vi "CFTS-Connections Dialog.vi"(2 "Parent VI":refnum<vi>) -> ()   [LabVIEW 2020]
doc: "Use this template to create a dialog box with event handling."
uses:
  epl-vi-lib/Utility VIs/Controls/KBackground Gradient/KBackground Gradient.xctl
  epl-vi-lib/Utility VIs/Controls/KTable/KTable.xctl
  epl-vi-lib/Connection VIs/Typedefs/CM-Endpoint.ctl
panel:
  in  "AO":u16(xcontrol)
  in  "AI":u16(xcontrol)
  in  "background":dbl(xcontrol)
  in  "Cancel":bool
  in  "OK":bool
  # "Connections"
  # "Outputs"
  # "Inputs"
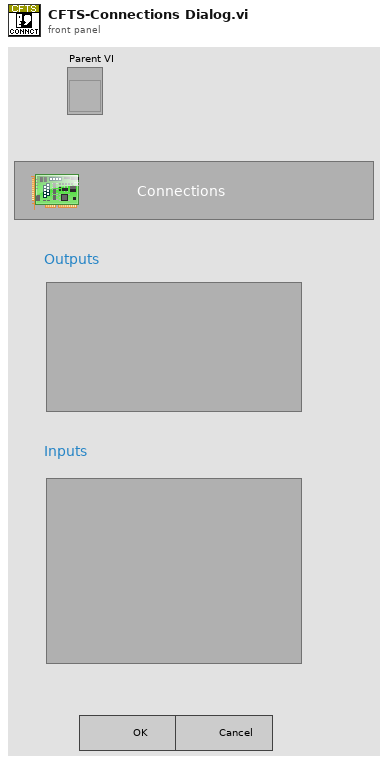
[diagram p1: front panel]
types:
  T1 = typedef "CM-Endpoint.ctl" = cluster{"Name":string, "Device":string}
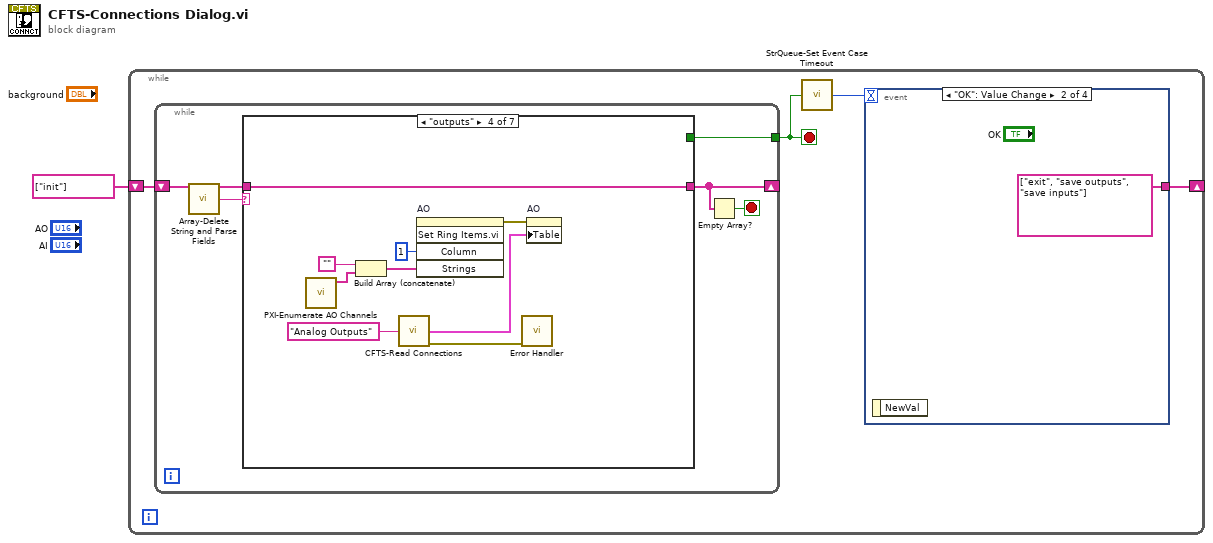
[diagram p0: block diagram]
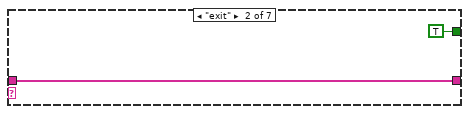
[diagram p3: hidden frame]
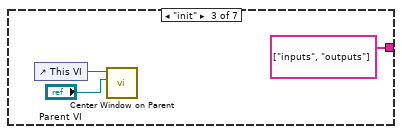
[diagram p4: hidden frame]
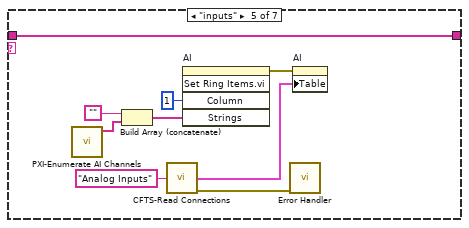
[diagram p5: hidden frame]
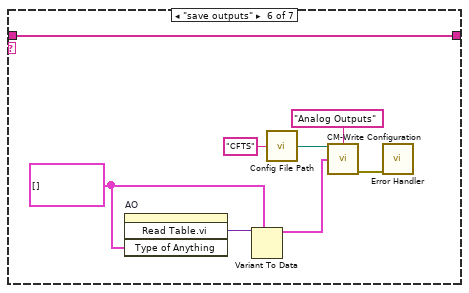
[diagram p6: hidden frame]
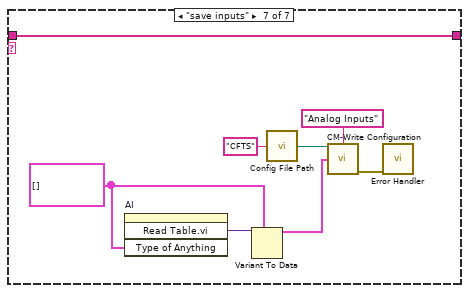
[diagram p7: hidden frame]
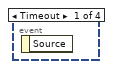
[diagram p8: hidden frame]
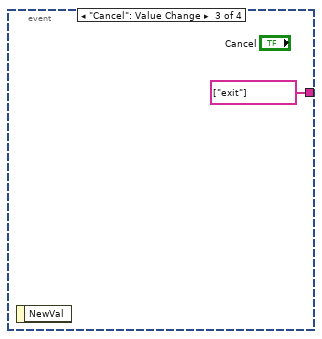
[diagram p9: hidden frame]
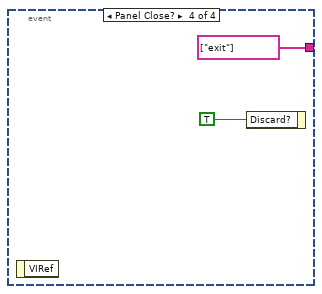
[diagram p10: hidden frame]
diagram:
  n1 = while {
    shift-right: [w2] -> _
    shift-left: string[] ["init"] -> [w3]
    stop <- w5 stop-if-true
    n2 = while {
      shift-right: [w11] -> _
      shift-left: w3 -> [w8]
      tunnel: [w9] -> w5
      stop <- w10 stop-if-true
      n3 = call "Array-Delete String and Parse Fields.vi"("Array in"=w8) -> ("Array out"=w7:string[], "Field 1"=w6:string)  [unwired: 10 in, 3 out]
      n4 = case shown="\"outputs\"" w6 {
        tunnel: w7 -> [w12 w14 _ w26 w35 w43 w51]
        tunnel: [w12 w14 string[] ["inputs", "outputs"] ("Array out") w26 w35 w43 w51] -> w11
        tunnel: [_ TRUE _ _ _ _ _] -> w9
        frame "", Default {
        }
        frame "exit" {
        }
        frame "init" {
          n5 = control-ref of="This VI"() -> (w16:refnum<vi>)
          n6 = call "Center Window on Parent.vi"("Parent VI"="Parent VI", "VI in"=w16) -> ()  [unwired: 8 in, 2 out]
        }
        frame "outputs" {
          n7 = call "PXI-Enumerate AO Channels.vi"() -> ("AO.PhysicalChans"=w23:tag[])  [unwired: 11 in]
          n8 = Build Array (concatenate)("", w23) -> (w21:string[])
          n9 = call "CFTS-Read Connections.vi"("Which"="Analog Outputs") -> ("endpoints"=w19:T1[], "error out"=w20:errorcluster)  [unwired: 13 in]
          n10 = invoke on="AO" class="KTable (strict)" method="Set Ring Items.vi"("Column"=1, "Strings"=w21) -> (error out=w25:errorcluster)  [unwired: 3 in, 4 out]
          n11 = call "Error Handler.vi"("error in (no error)"=w20) -> ()  [unwired: 13 in, 2 out]
          n12 = property on="AO" class="KTable (strict)"(error in=w25, "Table"=w19) -> ()  [unwired: 1 in, 2 out]
        }
        frame "inputs" {
          n13 = call "PXI-Enumerate AI Channels.vi"() -> ("AI.PhysicalChans"=w32:tag[])  [unwired: 11 in]
          n14 = Build Array (concatenate)("", w32) -> (w30:string[])
          n15 = call "CFTS-Read Connections.vi"("Which"="Analog Inputs") -> ("endpoints"=w28:T1[], "error out"=w29:errorcluster)  [unwired: 13 in]
          n16 = invoke on="AI" class="KTable (strict)" method="Set Ring Items.vi"("Column"=1, "Strings"=w30) -> (error out=w34:errorcluster)  [unwired: 3 in, 4 out]
          n17 = call "Error Handler.vi"("error in (no error)"=w29) -> ()  [unwired: 13 in, 2 out]
          n18 = property on="AI" class="KTable (strict)"(error in=w34, "Table"=w28) -> ()  [unwired: 1 in, 2 out]
        }
        frame "save outputs" {
          w40 = T1[] [] ("Array")
          n19 = invoke on="AO" class="KTable (strict)" method="Read Table.vi"("Type of Anything"=w40) -> ("Read Table.vi"=w41:variant)  [unwired: 3 in, 3 out]
          n20 = Variant To Data(type=w40, Variant=w41) -> (data=w38:T1[])  [unwired: 1 in, 1 out]
          n21 = call "Config File Path.vi"("AppName"="CFTS") -> ("Default config file name"=w39:path)
          n22 = call "CM-Write Configuration.vi"("Connection File Path"=w39, "Section"="Analog Outputs", "Endpoints"=w38) -> ("error out"=w36:errorcluster)  [unwired: 11 in, 1 out]
          n23 = call "Error Handler.vi"("error in (no error)"=w36) -> ()  [unwired: 13 in, 2 out]
        }
        frame "save inputs" {
          w48 = T1[] [] ("Array")
          n24 = invoke on="AI" class="KTable (strict)" method="Read Table.vi"("Type of Anything"=w48) -> ("Read Table.vi"=w49:variant)  [unwired: 3 in, 3 out]
          n25 = Variant To Data(type=w48, Variant=w49) -> (data=w46:T1[])  [unwired: 1 in, 1 out]
          n26 = call "Config File Path.vi"("AppName"="CFTS") -> ("Default config file name"=w47:path)
          n27 = call "CM-Write Configuration.vi"("Connection File Path"=w47, "Section"="Analog Inputs", "Endpoints"=w46) -> ("error out"=w44:errorcluster)  [unwired: 11 in, 1 out]
          n28 = call "Error Handler.vi"("error in (no error)"=w44) -> ()  [unwired: 13 in, 2 out]
        }
      }
      n29 = Empty Array?(array=w11) -> (empty?=w10:bool)
    }
    n30 = call "StrQueue-Set Event Case Timeout.vi"("Quit"=w5) -> ("timeout"=w4:i32)  [unwired: 14 in]
    n31 = event shown="[1] \"OK\": Value Change" {
      selector: _ -> [_ _ _ _]
      dyn-events: _ -> [_ _ _ _]
      timeout: w4 -> [_ _ _ _]
      tunnel: [_ string[] ["exit", "save outputs", "save inputs"] string[] ["exit"] string[] ["exit"]] -> w2
      event Timeout {
        n32 = event-data() -> ()  [unwired: 1 in, 1 out]
      }
      event "OK": Value Change {
        n33 = event-data() -> ()  [unwired: 1 in, 1 out]
      }
      event "Cancel": Value Change {
        n34 = event-data() -> ()  [unwired: 1 in, 1 out]
      }
      event Panel Close? {
        n35 = event-data() -> ()  [unwired: 1 in, 1 out]
        n36 = event-data("Discard?"=TRUE) -> ()  [unwired: 1 in, 1 out]
      }
    }
  }
